vi "Read Format string.vi"(8 "error in (no error)":errorcluster, 11 "Float D Element in":refnum<class "Float D Element.lvclass">) -> (0 "error out":errorcluster, 2 "Format string":string, 3 "Float D Element out":refnum<class "Float D Element.lvclass">)   [LabVIEW 2018, in "D Datagrid Library.lvlib" / "Float D Element.lvclass"]
uses:
  Float D Element.lvclass
  Floating point base/Floating point base.lvclass
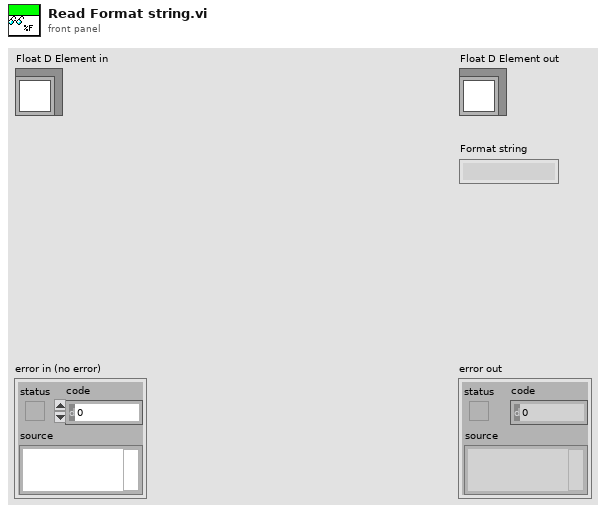
[diagram p1: front panel]
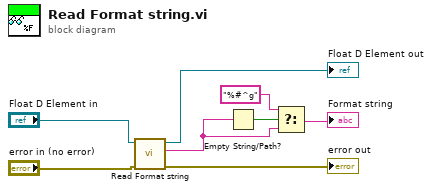
[diagram p0: block diagram]
diagram:
  n1 = call-parent "Read Format string.vi"("error in (no error)"="error in (no error)", "Floating point base in"="Float D Element in") -> ("error out"=→"error out":errorcluster, "Format string"=w6:string, "Floating point base out"=→"Float D Element out":refnum<class "Float D Element.lvclass">)  [unwired: 7 in]
  n2 = Empty String/Path?(string/path=w6) -> (empty?=w8:bool)
  n3 = Select(t="%#^g" ("format string"), s=w8, f=w6) -> (s? t:f=→"Format string":string)
